vi "sumo SIMPLES.vi"   [LabVIEW 2016]
uses:
  <vilib>/NXT/Subs/LVHSConnector.ctl
  <vilib>/NXT/LegoClasses/BrickReference/BrickReference.lvclass
  <vilib>/NXT/Block Support/NXT_ButtonSelector.ctl
  <vilib>/NXT/Block Support/NXT_InputPort.ctl
  <vilib>/NXT/Block Support/NXT_OutputPort.ctl
  <vilib>/NXT/Dual Mode Library/Waits/Wait_Num.vi
  <vilib>/NXT/Dual Mode Library/Sensors/EV3_Color_Reflect.vi
  <vilib>/NXT/Dual Mode Library/Sound/Tone.vi
  <vilib>/NXT/NXTIO Xnodes/NXTIONodeSubVIs/NXTMoveMotors.vi
  <vilib>/NXT/Dual Mode Library/Sensors/EV3_Ultrasonic_CM.vi
  <vilib>/NXT/Dual Mode Library/Sensors/readNXTButton.vi
  <vilib>/NXT/NXTIO Xnodes/AddressXNode/NXTIOAddress.xnode
  r2d2/sumobasico.lvrbt
  <vilib>/NXT/NXTIO Xnodes/NXTIOXNode/NXTIO.xnode
types:
  T1 = typedef "LVHSConnector.ctl" = refnum<class "BrickReference.lvclass">
  T2 = typedef "NXT_OutputPort.ctl" = u8
  T3 = typedef "NXT_InputPort.ctl" = u32
  T4 = typedef "NXT_ButtonSelector.ctl" = u16
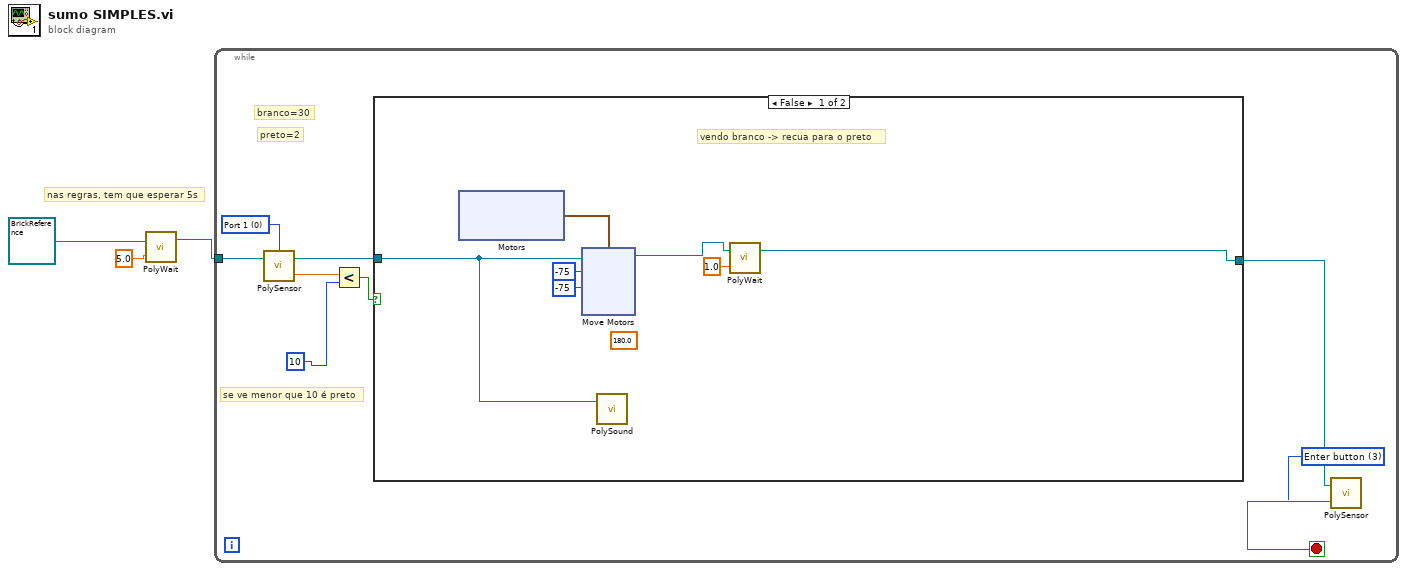
[diagram p0: block diagram]
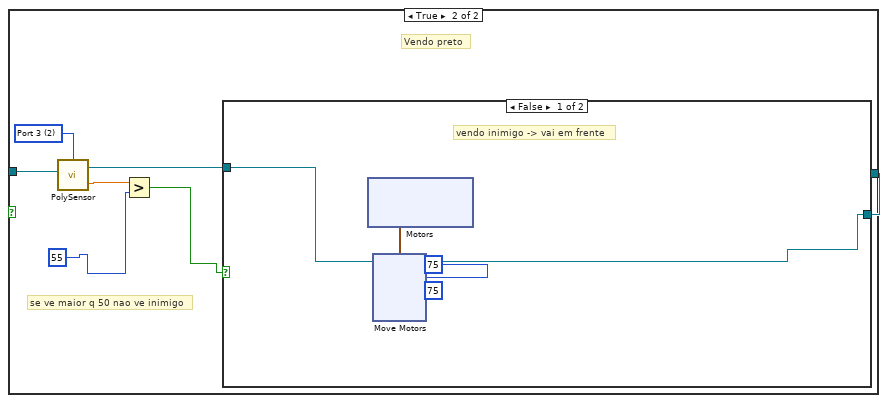
[diagram p2: hidden frame]
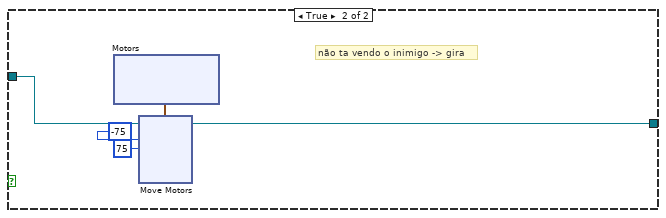
[diagram p3: hidden frame]
diagram:
  # "nas regras, tem que esperar 5s"
  n1 = call-poly <vilib>:"PolyWait.vi"("Time (1 sec)"=sgl 5.0, "NXT/EV3"=T1 refnum) -> ("NXT/EV3"=w1:T1)  [unwired: 2 in]
  n2 = while {
    tunnel: w1 -> [w5]
    stop <- w12 stop-if-true
    w11 = T3 0 items=["Port 1", "Port 2", "Port 3", "Port 4"] ("Port (Port 1)")
    w10 = T4 3 items=["Enter button"=3, "Left button"=2, "Right button"=1, "Up Button"=4, "Down Button"=5] ("Button (Enter button)")
    # "se ve menor que 10 é preto"
    # "preto=2"
    # "branco=30"
    n3 = call-poly <vilib>:"PolySensor.vi"("NXT/EV3"=w5, "Port (Port 1)"=w11) -> ("Scaled Value"=w9:sgl, "NXT/EV3"=w7:T1)  [unwired: 1 in]
    n4 = Less?(x=w9, y=10) -> (x < y?=w6:bool)
    n5 = case shown="False" w6 {
      tunnel: w7 -> [w14 w31]
      tunnel: [w13 w29] -> w4
      frame False {
        (unwired) sgl 180.0 ("Time (1 sec)")
        # "vendo branco -> recua para o preto"
        n6 = xnode "Motors"() -> ("Motor"=w17:cluster{"Port":T2, "Port":T2})
        n7 = xnode "Move Motors"("Power/Speed 2"=i8 -75, "Power/Speed 1"=i8 -75, "Motors"=w17, "NXT/EV3"=w14) -> ("NXT/EV3"=w15:T1)
        n8 = call-poly <vilib>:"PolySound.vi"("NXT/EV3"=w14) -> ()  [unwired: 3 in, 1 out]
        n9 = call-poly <vilib>:"PolyWait.vi"("Time (1 sec)"=sgl 1.0, "NXT/EV3"=w15) -> ("NXT/EV3"=w13:T1)  [unwired: 2 in]
      }
      frame True {
        w33 = T3 2 items=["Port 1", "Port 2", "Port 3", "Port 4"] ("Port (Port 1)")
        # "Vendo preto"
        # "se ve maior q 50 nao ve inimigo"
        n10 = call-poly <vilib>:"PolySensor.vi"("NXT/EV3"=w31, "Port (Port 1)"=w33) -> ("Centimeters"=w35:sgl, "NXT/EV3"=w30:T1)  [unwired: 1 in]
        n11 = Greater?(x=w35, y=55) -> (0:w32:bool)
        n12 = case shown="False" w32 {
          tunnel: w30 -> [w37 w51]
          tunnel: [w36 w50] -> w29
          frame False {
            # "vendo inimigo -> vai em frente"
            n13 = xnode "Motors"() -> ("Motor"=w40:cluster{"Port":T2, "Port":T2})
            n14 = xnode "Move Motors"("Power/Speed 2"=i8 75, "Power/Speed 1"=i8 75, "Motors"=w40, "NXT/EV3"=w37) -> ("NXT/EV3"=w36:T1)
          }
          frame True {
            # "não ta vendo o inimigo -> gira"
            n15 = xnode "Motors"() -> ("Motor"=w54:cluster{"Port":T2, "Port":T2})
            n16 = xnode "Move Motors"("Power/Speed 2"=i8 75, "Power/Speed 1"=i8 -75, "Motors"=w54, "NXT/EV3"=w51) -> ("NXT/EV3"=w50:T1)
          }
        }
      }
    }
    n17 = call-poly <vilib>:"PolySensor.vi"("Button (Enter button)"=w10, "NXT/EV3"=w4) -> ("Yes/No"=w12:bool)  [unwired: 1 in, 1 out]
  }
